vi "SENSORES Values JSON.vi"(5 "Boolean":bool, 7 "JSON  HumeRel":refnum<class "JSON Object.lvclass">=refnum, 8 "error in":errorcluster, 9 "tempPanel":refnum<class "JSON Object.lvclass">=refnum, 10 "tempAmb":refnum<class "JSON Object.lvclass">=refnum, 11 "JSON PAR":refnum<class "JSON Object.lvclass">=refnum) -> (0 "error out":errorcluster, 3 "JSON Object out":refnum<class "JSON Object.lvclass">)   [LabVIEW 2015]
uses:
  <vilib>/addons/JSON API/JSON Object/Set Object Item by name.vi
  <vilib>/addons/JSON API/JSON Object/JSON Object.lvclass
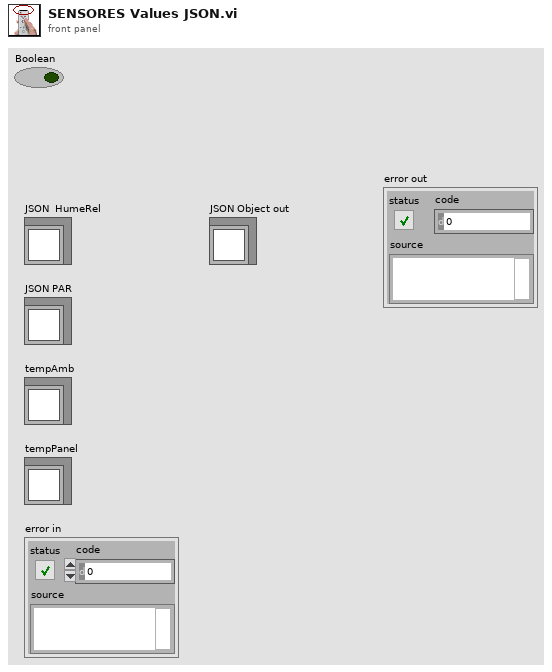
[diagram p1: front panel]
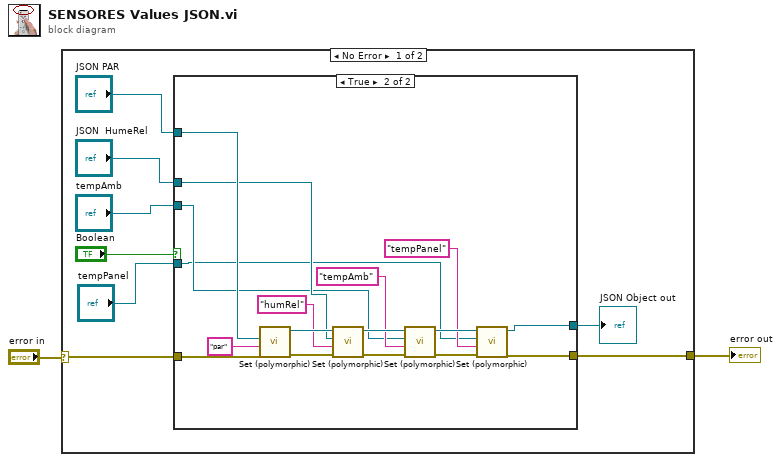
[diagram p0: block diagram]
diagram:
  n1 = case shown="No Error" "error in" {
    selector: "error in" -> [w3 w29]
    tunnel: [w5 w29] -> w2
    frame No Error {
      n2 = case shown="True" "Boolean" {
        tunnel: [_ w21] -> w6
        tunnel: "JSON PAR" -> [_ w17]
        tunnel: "JSON  HumeRel" -> [_ w16]
        tunnel: "tempAmb" -> [_ w15]
        tunnel: "tempPanel" -> [_ w14]
        tunnel: w3 -> [w11 w13]
        tunnel: [w11 w12] -> w5
        frame False {
        }
        frame True {
          n3 = call-poly <vilib>:"Set (polymorphic).vi"("error in (no error)"=w13, "name"="par", "Value"=w17) -> ("error out"=w20:errorcluster, "JSON Object out"=w27:refnum<class "JSON Object.lvclass">)  [unwired: 6 in, 1 out]
          n4 = call-poly <vilib>:"Set (polymorphic).vi"("error in (no error)"=w20, "name"="humRel", "Value"=w16, "JSON Object in"=w27) -> ("error out"=w19:errorcluster, "JSON Object out"=w25:refnum<class "JSON Object.lvclass">)  [unwired: 5 in, 1 out]
          n5 = call-poly <vilib>:"Set (polymorphic).vi"("error in (no error)"=w19, "name"="tempAmb", "Value"=w15, "JSON Object in"=w25) -> ("error out"=w18:errorcluster, "JSON Object out"=w23:refnum<class "JSON Object.lvclass">)  [unwired: 5 in, 1 out]
          n6 = call-poly <vilib>:"Set (polymorphic).vi"("error in (no error)"=w18, "name"="tempPanel", "Value"=w14, "JSON Object in"=w23) -> ("error out"=w12:errorcluster, "JSON Object out"=w21:refnum<class "JSON Object.lvclass">)  [unwired: 5 in, 1 out]
        }
      }
      "JSON Object out" <- w6
    }
    frame Error {
    }
  }
  "error out" <- w2
